vi "Main_6a original.vi"() -> ()   [LabVIEW 2020]
uses:
  0c0f8bb7-c444-485a-b807-04b59ab5f06f.vi
panel:
  out "Position of marker":i32
  in  "Example 5":string="zcfzfwzzqfrljwzlrfnpqdbhtmscgvjw"
  in  "Example 4":string="nznrnfrfntjfmvfwmzdfjlvtqnbhcprsg"
  in  "Example 3":string="nppdvjthqldpwncqszvftbrmjlhg"
  in  "Example 2":string="bvwbjplbgvbhsrlpgdmjqwftvncz"
  in  "Puzzle":string="plhlsssjsrscspsffmrffwvfvrvvmbbnjnrnrfnndlnlznlznlnccdbbhvbvgvmvzmzvmzmbbrcclsslzslzzsztzftzzhggnjgnjnhnmnqnqqfdfnnrwnwsnwwvgvqqgpptvtrvvfmmzjzmmjssmwsmmhzzvvwzwcwrcrllpbppdgdvvwqvvsnsrnsncnwntnggwqgqhqrqprqrddjvddqsqhshchfffzddswdsshhcnhnqqfjffvlvwvssdqqwrwvrvhrvrzzgwggcjcgclcwchhzvzmzrrjwjqwwvbwwrmmvmpmzpzgpgsghgrrtmmlfmmnzzmpzzvmvjjsqqshqshsqqgtqggpvvrtttwbbhnbnlbnlnhnthtjhjshhrmrjjlclpprmrnrsrwrbwrwwjnwnbwbhbmbggdbgghllcvlvddzbdbdvdwvdvjvqvcvczvcvclvvrggrngrrwcwbcczgghnhznhnttbcbvcvttrrpbrppndppvvvgvtgvvhfvhhttppjmjllznlnldnldlwlnwlnlttgzzcfcggwmgmqgmmshmhqqdfqfpfqppprzrhrnrhnrrtsrrgpgnpng..."
  in  "Example":string="mjqjpqmgbljsphdztnvjfqwrcgsmlb"
  # "--- Day 6: Tuning Trouble ---\nThe preparations are finally complete; you and the Elves leave camp on foot and begin to make your way toward the star fruit grove.\n\nAs you move through the dense undergrowth, one of the Elves gives you a handheld device. He says that it has many fancy features, but the most important one to set up right now is the communication system.\n\nHowever, because he's heard you have significant experience dealing with signal-based systems, he convinced the other Elves that it would be okay to give you their one malfunctioning device - surely you'll have no problem fixing it.\n\nAs if inspired by comedic timing, the device emits a few colorful sparks.\n\nTo be able to communicate with the Elves, the device needs to lock on to their signal. The signal is a series of seemingly-random characters that the device receives one at a time.\n\nTo fix the communication system, you need to add a subroutine to the device that detects a start-of-packet marker in the datastream. In the protocol being used by the Elves, the start of a packet is indicated by a sequence of four characters that are all different.\n\nThe device will send your subroutine a datastream buffer (your puzzle input); your subroutine needs to identify the first position where the four most recently received characters were all different. Specifically, it needs to report the number of characters from the beginning of the buffer to the end of the first such four-character marker.\n\nFor example, suppose you receive the following datastream buffer:\n\nmjqjpqmgbljsphdztnvjfqwrcgsmlb\nAfter the first three characters (mjq) have been received, there haven't been enough characters received yet to find the marker. The first time a marker could occur is after the fourth character is received, making the most recent four characters mjqj. Because j is repeated, this isn't a marker.\n\nThe first time a marker appears is after the seventh character arrives. Once it does, the last four characters received are jpqm, which are all different. In this case, your subroutine should report the value 7, because the first start-of-packet marker is complete after 7 characters have been processed.\n\nHere are a few more examples:\n\nbvwbjplbgvbhsrlpgdmjqwftvncz: first marker after character 5\nnppdvjthqldpwncqszvftbrmjlhg: first marker after character 6\nnznrnfrfntjfmvfwmzdfjlvtqnbhcprsg: first marker after character 10\nzcfzfwzzqfrljwzlrfnpqdbhtmscgvjw: first marker after character 11\nHow many characters need to be processed before the first start-of-packet marker is detected?"
  # "1287"
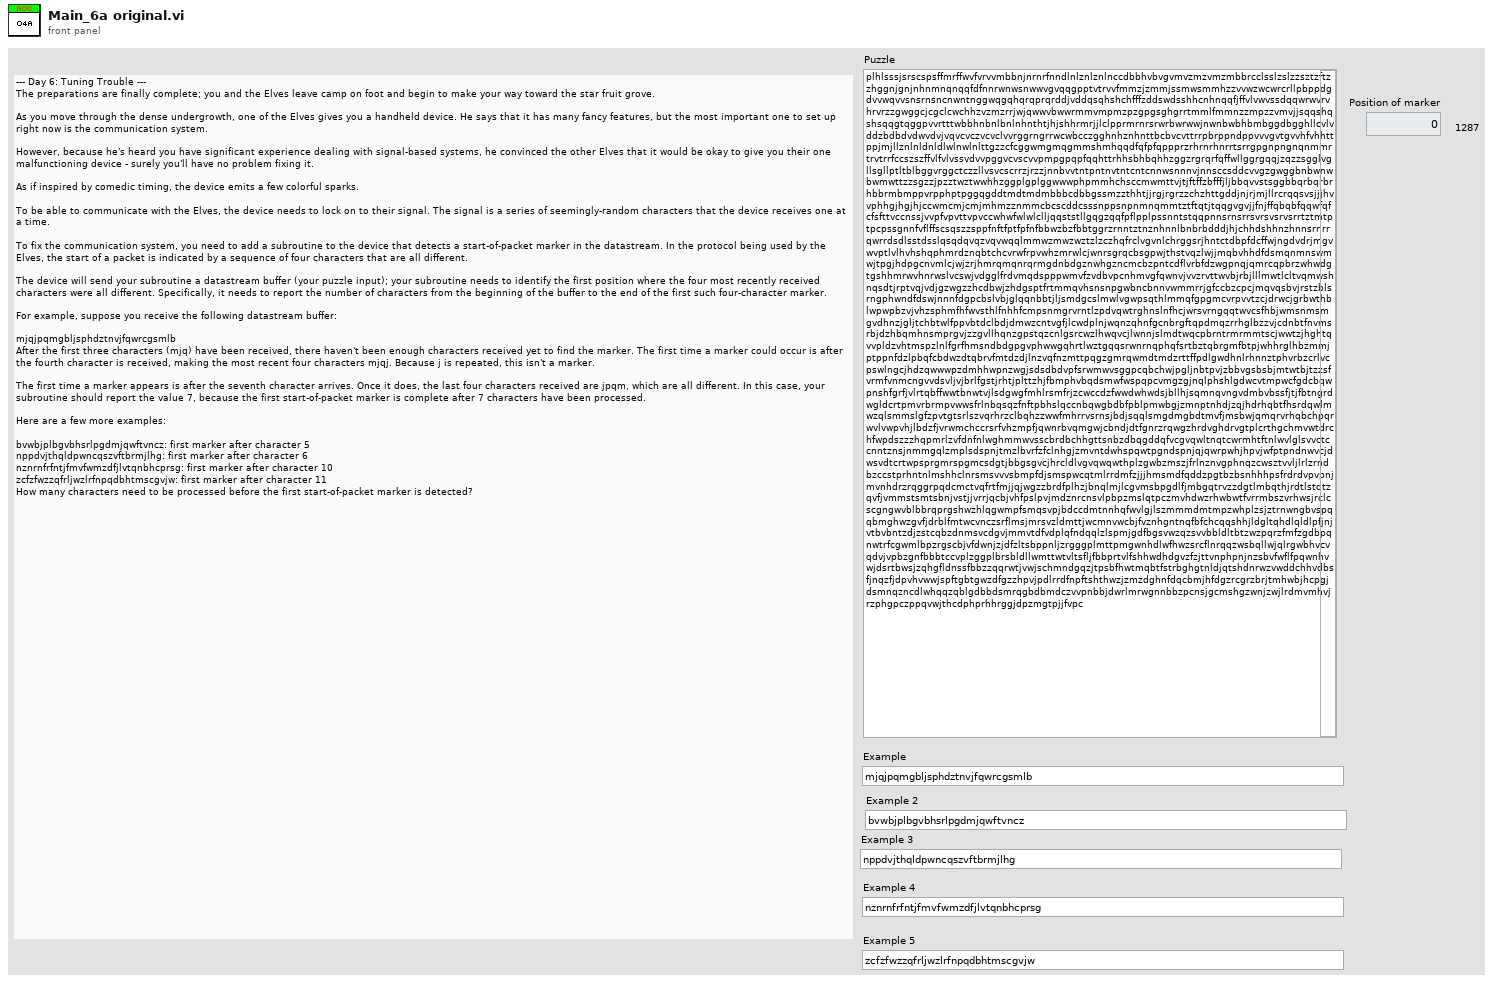
[diagram p1: front panel]
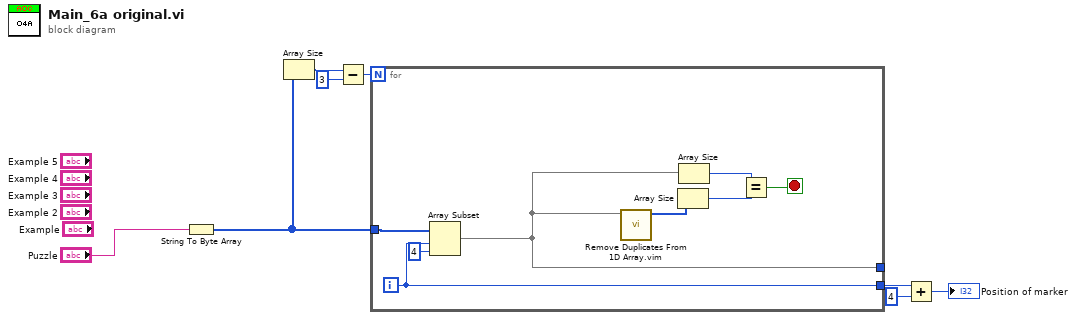
[diagram p0: block diagram]
diagram:
  n1 = String To Byte Array(string="Puzzle") -> (unsigned byte array=w5:u8[])
  n2 = Array Size(array=w5) -> (size(s)=w8:i32)
  n3 = Subtract(x=w8, y=3) -> (x-y=w6:i32)
  n4 = for {
    N: w6 -> [_]
    tunnel: w5 -> [w16]
    tunnel: [w11] -> _
    tunnel: [w12] -> w4
    i -> [w12]
    stop <- w13 stop-if-true
    n5 = Array Subset(array=w16, index=w12, length=4) -> (w11:u8[])
    n6 = call "Remove Duplicates From 1D Array.vim"("array"=w11) -> ("array with duplicates removed"=w10:u8[])  [unwired: 10 in]
    n7 = Array Size(array=w10) -> (size(s)=w9:i32)
    n8 = Array Size(array=w11) -> (size(s)=w14:i32)
    n9 = Equal?(x=w14, y=w9) -> (x = y?=w13:bool)
  }
  n10 = Add(x=w4, y=4) -> (x+y=→"Position of marker":i32)
